vi "Flywheel_Execute.vi"() -> ()   [LabVIEW 2020]
uses:
  Globals/Flywheel_Globals.vi
  Globals/Sensor_Values.vi
  Utility VIs/Basic_Motor_Modes.ctl
panel:
  in  "array 2":dbl[][](array[numeric])
  in  "array":dbl[][](array[numeric])
  out "added Area":dbl=-0.27951836585998535
  in  "Camera Area D":dbl=17.0
  in  "Default_Flywheel_Speed":dbl=4750.0
  in  "Flywheel_MaxSpeed(RPM)":dbl=4900.0
  out "Camera_Area":dbl=1.2052602767944336
  out "Error":cluster{dbl, dbl}(graph)
  out "Spun-Up":bool
  out "Error":dbl
  in  "Acceptable_error":dbl=200.0
  # "Click here to set min"
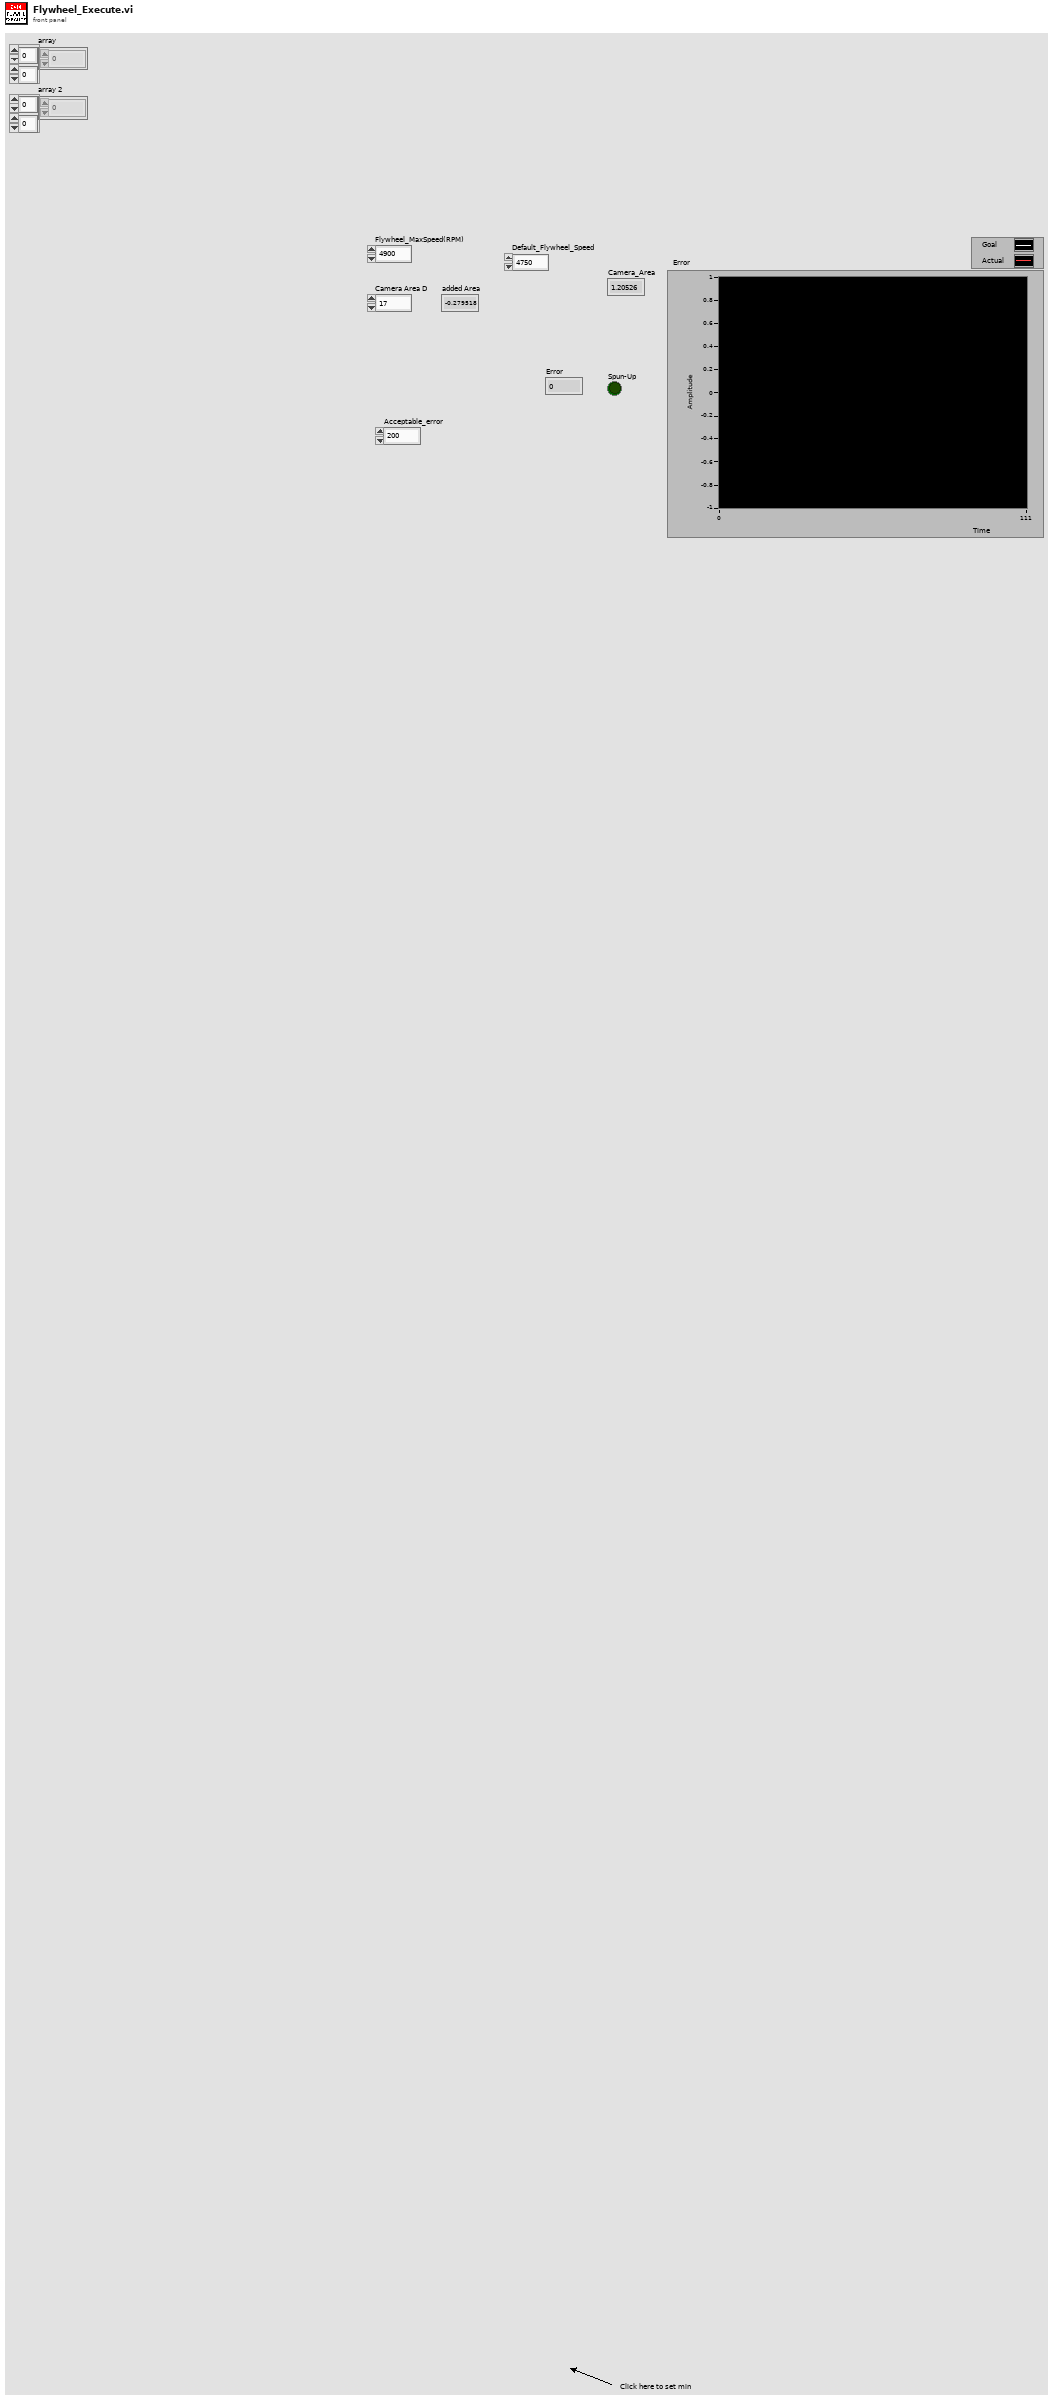
[diagram p1: front panel]
types:
  T1 = typedef "Basic_Motor_Modes.ctl" = enum16{"Percent_Voltage", "Speed_Control", "Position_Control", "Current"}
  T2 = typedef "Flywheel_Cluster.ctl" = cluster{"Flywheel_Throttle":dbl, "Flywheel_Control_State":T3, "Parameter_1":dbl, "Parameter_2":dbl, "Auto_Notifier":refnum<notifier>, "Step":dbl, "Flywheel_Velocity_Goal":dbl, "Flywheel_On ":bool}
  T3 = typedef "Flywheel_States.ctl" = enum16{"No-Op", "Percent_Voltage", "Speed_Control_Manual", "Speed_Control_Auto", "Command_SpinUp", "Command_SpinUpAuto"}
  T4 = cluster{"Flywheel_Output":dbl, "Flywheel_Velocity(RPM)":dbl}
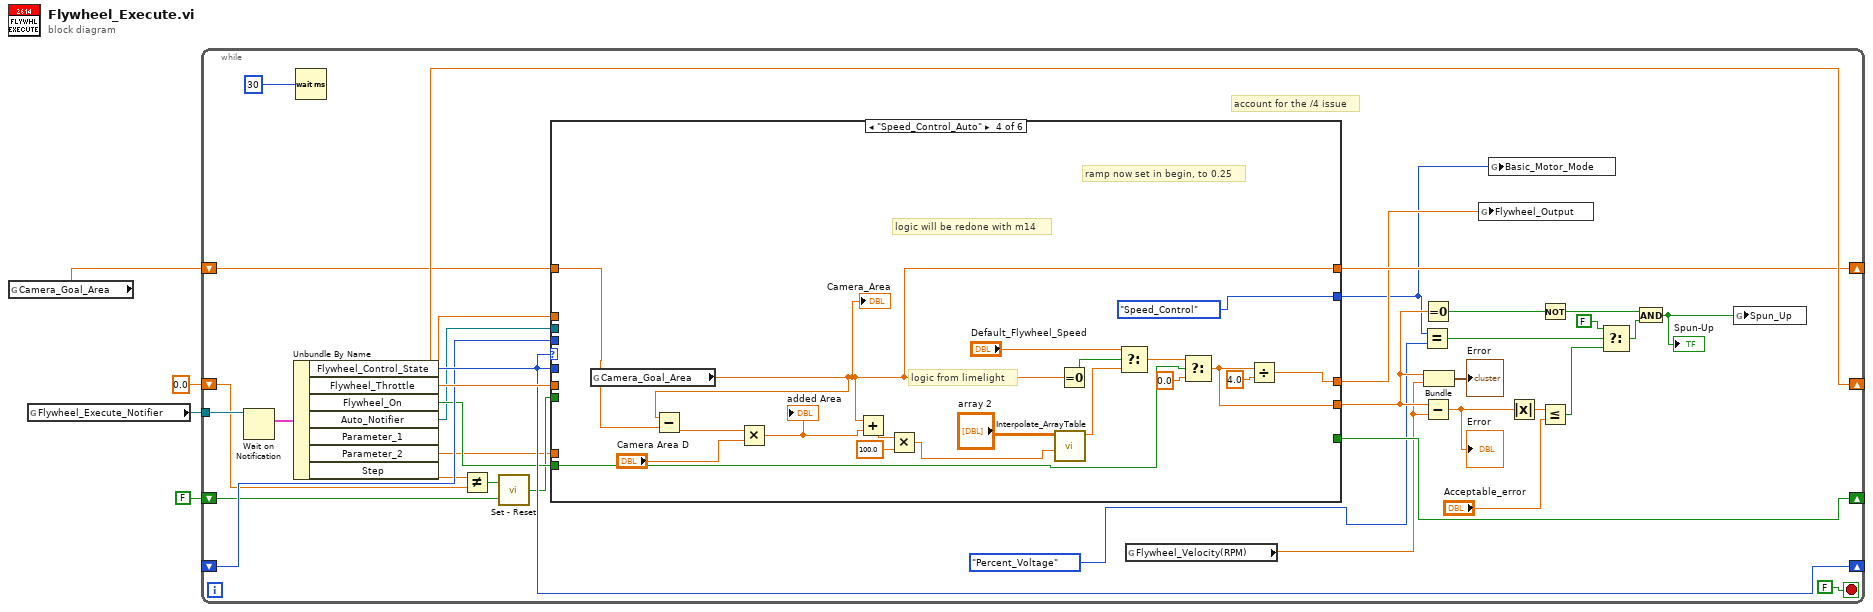
[diagram p0: block diagram]
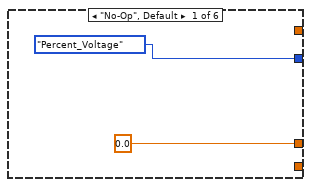
[diagram p2: hidden frame]
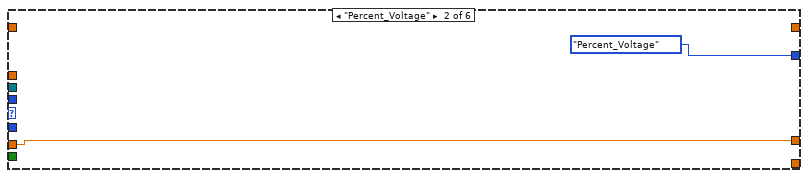
[diagram p3: hidden frame]
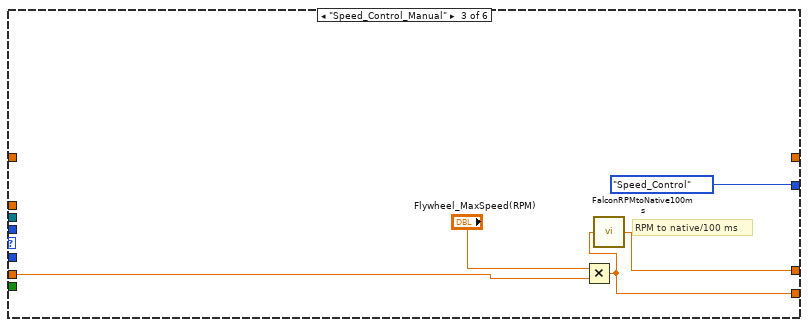
[diagram p4: hidden frame]
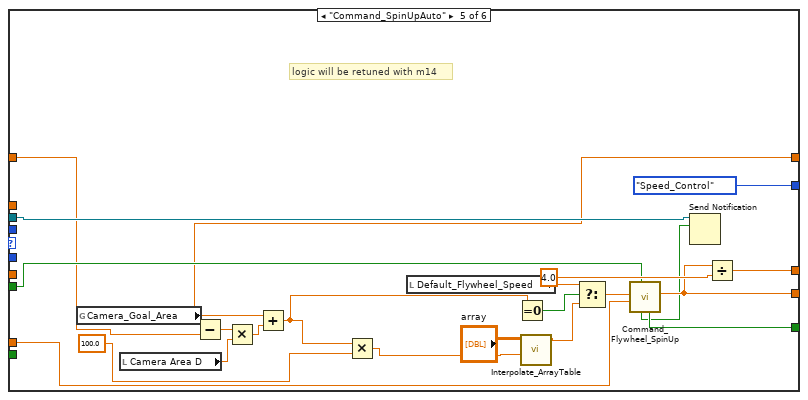
[diagram p5: hidden frame]
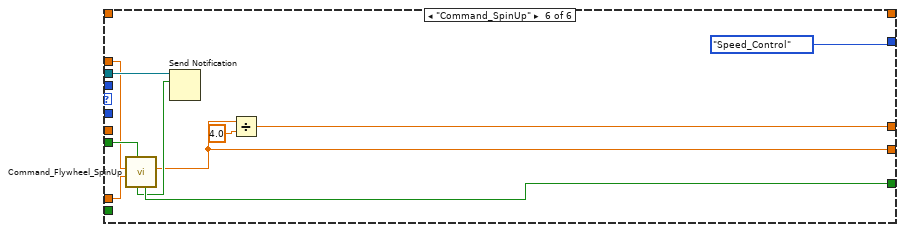
[diagram p6: hidden frame]
diagram:
  n1 = global read "Sensor_Values.vi" "Camera_Goal_Area"() -> (w1:dbl)
  n2 = global read "Flywheel_Globals.vi" "Flywheel_Execute_Notifier"() -> (w4:refnum<notifier>)
  n3 = while {
    tunnel: w4 -> [w38]
    shift-right: [w34] -> _
    shift-left: _ -> [w33]
    shift-right: [w12] -> _
    shift-left: 0.0 ("Step") -> [w11]
    shift-right: [w17] -> _
    shift-left: FALSE ("Reint") -> [w18]
    shift-right: [w9] -> _
    shift-left: w1 -> [w10]
    stop <- FALSE stop-if-true
    # "account for the /4 issue"
    n4 = Wait on Notification(notifier=w38) -> (notification=w37:T2)  [unwired: 3 in, 3 out]
    n5 = Unbundle By Name(w37) -> ("Flywheel_Control_State"=w34:T3, "Flywheel_Throttle"=w36:dbl, "Flywheel_On"=w22:bool, "Auto_Notifier"=w16:refnum<notifier>, "Parameter_1"=w15:dbl, "Parameter_2"=w14:dbl, "Step"=w12:dbl)
    n6 = Wait (ms)(milliseconds to wait=u32 30) -> ()  [unwired: 1 out]
    n7 = Not Equal?(x=w12, y=w11) -> (x != y?=w13:bool)
    n8 = call "Set - Reset.vi"("Reset"=w18, "Set"=w13) -> ("Output"=w19:bool)
    n9 = case shown="\"Speed_Control_Auto\"" w34 {
      tunnel: [0.0 ("Flywheel_Throttle") w43 w44 w67 w88 w93] -> w8
      tunnel: w36 -> [_ w43 w48 _ _ _]
      tunnel: w34 -> [_ _ _ _ _ _]
      tunnel: w33 -> [_ _ _ _ _ _]
      tunnel: [_ _ w45 w66 w83 w91] -> w24
      tunnel: w22 -> [_ _ _ w65 _ _]
      tunnel: w19 -> [_ _ _ _ w81 w99]
      tunnel: [_ _ _ _ w80 w98] -> w17
      tunnel: w16 -> [_ _ _ _ w79 w97]
      tunnel: w15 -> [_ _ _ _ _ w95]
      tunnel: w14 -> [_ _ _ _ w82 w94]
      tunnel: w10 -> [_ _ _ w57 w70 _]
      tunnel: [_ _ _ w52 w74 _] -> w9
      tunnel: [Basic_Motor_Modes."Percent_Voltage" ("Motor_Mode") Basic_Motor_Modes."Percent_Voltage" ("Motor_Mode") Basic_Motor_Modes."Speed_Control" ("Motor_Mode") Basic_Motor_Modes."Speed_Control" ("Motor_Mode") Basic_Motor_Modes."Speed_Control" ("Motor_Mode") Basic_Motor_Modes."Speed_Control" ("Motor_Mode")] -> w6
      frame "No-Op", Default {
      }
      frame "Percent_Voltage" {
      }
      frame "Speed_Control_Manual" {
        # "RPM to native/100 ms"
        n10 = Multiply(x="Flywheel_MaxSpeed(RPM)", y=w48) -> (x*y=w45:dbl)
        n11 = call "FalconRPMtoNative100ms.vi"("RPM"=w45) -> ("raw sensor units / 100 ms"=w44:dbl)  [unwired: 4 in]
      }
      frame "Speed_Control_Auto" {
        # "logic will be redone with m14"
        # "ramp now set in begin, to 0.25"
        # "logic from limelight"
        n12 = global read "Sensor_Values.vi" "Camera_Goal_Area"() -> (w52:dbl)
        "Camera_Area" <- w52
        n13 = Subtract(x=w52, y=w57) -> (x-y=w56:dbl)
        n14 = Multiply(x=w56, y="Camera Area D") -> (x*y=w51:dbl)
        "added Area" <- w51
        n15 = Add(x=w52, y=w51) -> (x+y=w53:dbl)
        n16 = Multiply(x=w53, y=100.0) -> (x*y=w58:dbl)
        n17 = call "Interpolate_ArrayTable.vi"("Desired_Distance"=w58, "array"="array 2") -> ("RPM"=w59:dbl)  [unwired: 9 in]
        n18 = Equal To 0?(x=w52) -> (x = 0?=w62:bool)
        n19 = Select(t="Default_Flywheel_Speed", s=w62, f=w59) -> (s? t:f=w60:dbl)
        n20 = Select(t=w60, s=w65, f=0.0) -> (s? t:f=w66:dbl)
        n21 = Divide(x=w66, y=4.0) -> (x/y=w67:dbl)
      }
      frame "Command_SpinUpAuto" {
        # "logic will be retuned with m14"
        n22 = global read "Sensor_Values.vi" "Camera_Goal_Area"() -> (w74:dbl)
        n23 = local read "Camera Area D"() -> (w71:dbl)
        n24 = Subtract(x=w74, y=w70) -> (x-y=w73:dbl)
        n25 = Multiply(x=w73, y=w71) -> (x*y=w72:dbl)
        n26 = Add(x=w74, y=w72) -> (x+y=w75:dbl)
        n27 = Multiply(x=w75, y=100.0) -> (x*y=w76:dbl)
        n28 = local read "Default_Flywheel_Speed"() -> (w85:dbl)
        n29 = Equal To 0?(x=w75) -> (x = 0?=w86:bool)
        n30 = call "Interpolate_ArrayTable.vi"("Desired_Distance"=w76, "array"="array") -> ("RPM"=w77:dbl)  [unwired: 9 in]
        n31 = Select(t=w85, s=w86, f=w77) -> (s? t:f=w84:dbl)
        n32 = call "Command_Flywheel_SpinUp.vi"("Startup"=w81, "Timeout"=w82, "Speed"=w84) -> ("Flywheel_Output"=w83:dbl, "Reint"=w80:bool, "Completed"=w78:bool)  [unwired: 6 in]
        n33 = Send Notification(notification=w78, notifier=w79) -> ()  [unwired: 1 in, 2 out]
        n34 = Divide(x=w83, y=4.0) -> (x/y=w88:dbl)
      }
      frame "Command_SpinUp" {
        n35 = call "Command_Flywheel_SpinUp.vi"("Startup"=w99, "Timeout"=w94, "Speed"=w95) -> ("Flywheel_Output"=w91:dbl, "Reint"=w98:bool, "Completed"=w96:bool)  [unwired: 6 in]
        n36 = Send Notification(notification=w96, notifier=w97) -> ()  [unwired: 1 in, 2 out]
        n37 = Divide(x=w91, y=4.0) -> (x/y=w93:dbl)
      }
    }
    n38 = global read "Sensor_Values.vi" "Flywheel_Velocity(RPM)"() -> (w5:dbl)
    n39 = Equal?(x=w6, y=Basic_Motor_Modes."Percent_Voltage" ("Motor_Mode")) -> (x = y?=w30:bool)
    n40 = Equal To 0?(x=w24) -> (x = 0?=w27:bool)
    n41 = Subtract(x=w24, y=w5) -> (x-y=w25:dbl)
    "Error" <- w25
    n42 = Bundle("Flywheel_Output"=w24, "Flywheel_Velocity(RPM)"=w5) -> (→"Error":T4)  [unwired: 1 in]
    n43 = global write "Flywheel_Globals.vi" "Flywheel_Output"(w8) -> ()
    n44 = global write "Flywheel_Globals.vi" "Basic_Motor_Mode"(w6) -> ()
    n45 = Absolute Value(x=w25) -> (abs(x)=w32:dbl)
    n46 = Not(x=w27) -> (.not. x?=w26:bool)
    n47 = Less Or Equal?(x=w32, y="Acceptable_error") -> (x <= y?=w28:bool)
    n48 = Select(t=FALSE, s=w30, f=w28) -> (s? t:f=w21:bool)
    n49 = And(x=w26, y=w21) -> (x .and. y?=w20:bool)
    "Spun-Up" <- w20
    n50 = global write "Flywheel_Globals.vi" "Spun_Up"(w20) -> ()
  }
